vi "ws_mining search for scenario.vi"(6 "User":T3, 7 "httpRequestID":u32, 8 "error in (no error)":errorcluster, 10 "GET (empty)":T1, 11 "Connection Refnum":T2) -> (0 "error out":errorcluster, 1 "Template Keys":T1, 2 "Template":string, 3 "Connection Refnum":T2)   [LabVIEW 2011]
uses:
  server/database/Users/User Record.ctl
  <vilib>/addons/internet/utils/keyedarr.llb/Keyed Array.ctl
  SI.LIB/ODBC/SQL Controls/Connection Refnum.ctl
  <vilib>/addons/internet/utils/strutil.llb/Case Matching.ctl
  <vilib>/wsapi/NI_WebServices.lvlib
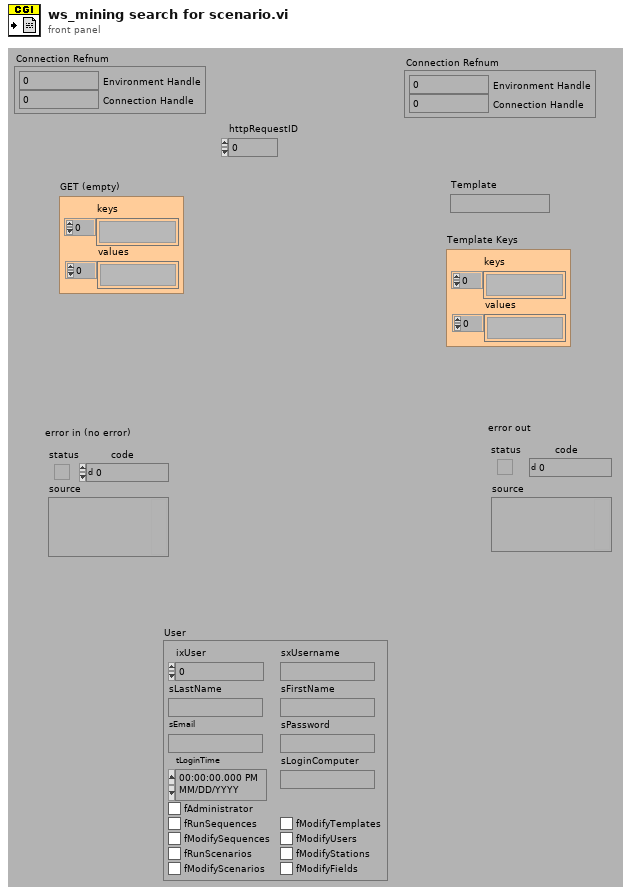
[diagram p1: front panel]
types:
  T1 = typedef "Keyed Array.ctl" = cluster{"keys":string[], "values":string[]}
  T2 = typedef "Connection Refnum.ctl" = cluster{"Environment Handle":i32, "Connection Handle":i32}
  T3 = typedef "User Record.ctl" = cluster{"ixUser":i32, "sxUsername":string, "sLastName":string, "sFirstName":string, "sEmail":string, "sPassword":string, "tLoginTime":timestamp, "sLoginComputer":string, "fAdministrator":bool, "fRunSequences":bool, "fModifySequences":bool, "fRunScenarios":bool, "fModifyScenarios":bool, "fModifyTemplates":bool, "fModifyUsers":bool, "fModifyStations":bool, "fModifyFields":bool}
  T4 = typedef "Case Matching.ctl" = enum16{"a != A", "a == A", "system"}
  T5 = typedef "Scenario Record.ctl" = cluster{"ixScenario":i32, "tCreated":timestamp, "tModified":timestamp, "sxUsername":string, "sModifiedBy":string, "sxScenarioId":string, "sDescription":string, "sLogic":string, "sResultFieldsCSV":string, "sTemplatesCSV":string, "fAutoRunReports":bool, "fSortByTemplates":bool, "fCombinePDF":bool, "Conditions":T6[]}
  T6 = typedef "Condition Record.ctl" = cluster{"iConditionIndex":i32, "sxFieldId":string, "nOperator":T7, "sMatchValue":string}
  T7 = typedef "Condition Operators.ctl" = enum16{"equal (=)", "not equal (\\u2260)", "less than (<)", "less than or equal (\\u2264)", "greater than (>)", "greater than or equal (\\u2265)", "contains", "does not contain"}
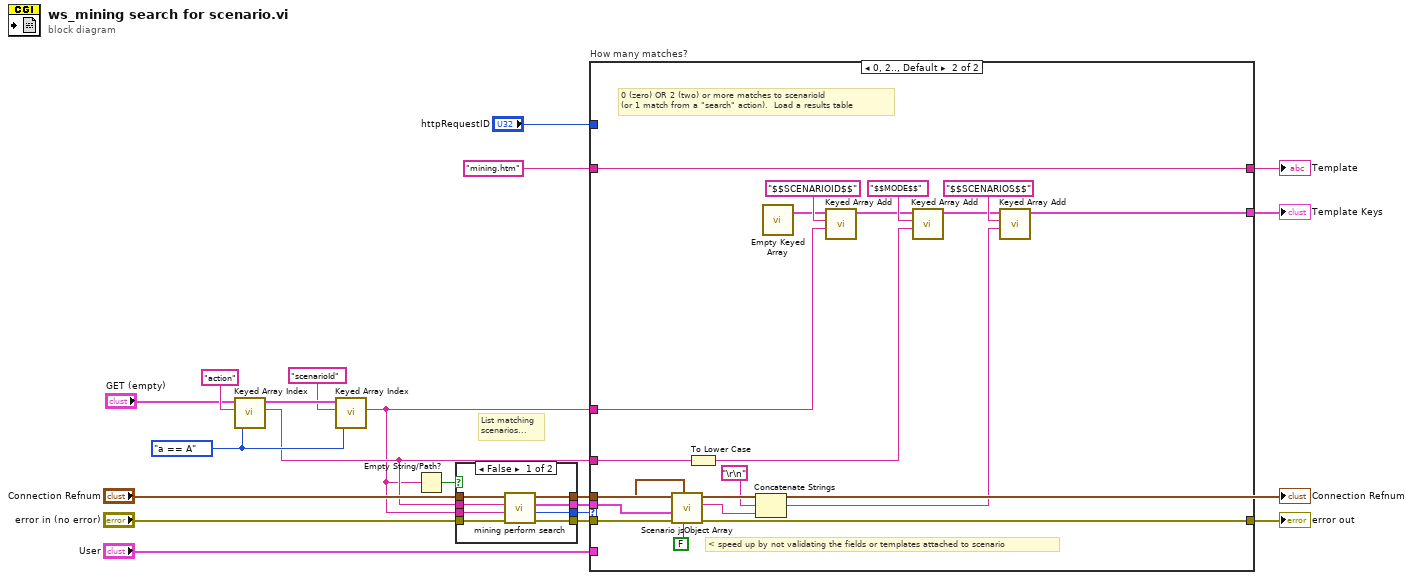
[diagram p0: block diagram]
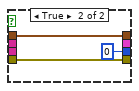
[diagram p2: hidden frame]
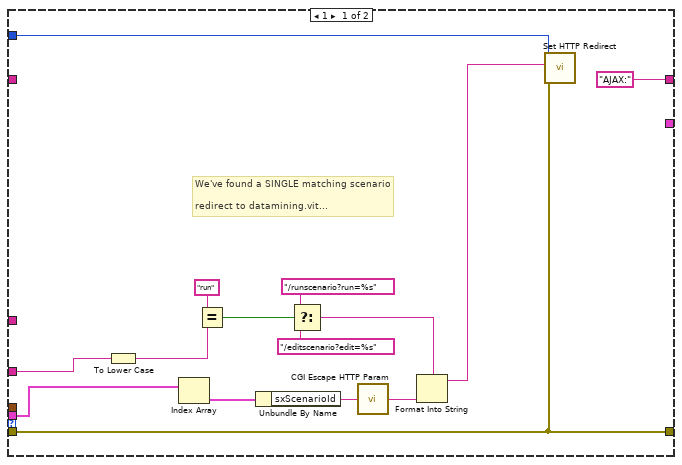
[diagram p3: hidden frame]
diagram:
  w8 = Case_Matching."a == A" ("case matching (sensitive)")
  # "List matching\nscenarios..."
  n1 = call <vilib>:"Keyed Array Index.vi"("case matching (sensitive)"=w8, "key"="action", "array in"="GET (empty)") -> ("value"=w7:string, "duplicate array"=w10:T1)  [unwired: 1 in, 2 out]
  n2 = call <vilib>:"Keyed Array Index.vi"("case matching (sensitive)"=w8, "key"="scenarioId", "array in"=w10) -> ("value"=w4:string)  [unwired: 1 in, 3 out]
  n3 = Empty String/Path?(string/path=w4) -> (empty?=w3:bool)
  n4 = case shown="False" w3 {
    tunnel: "error in (no error)" -> [w28 w30]
    tunnel: "Connection Refnum" -> [w27 w31]
    tunnel: [w26 w31] -> w2
    tunnel: [w25 _] -> w14
    tunnel: [w24 w30] -> w13
    tunnel: w7 -> [w23 _]
    tunnel: [w22 0 ("Matching Results")] -> w5
    tunnel: w4 -> [w21 _]
    frame False {
      n5 = call "mining perform search.vi"("error in (no error)"=w28, "sxScenarioId (\"\")"=w21, "Action (\"Search\")"=w23, "Connection Refnum"=w27) -> ("error out"=w24:errorcluster, "Matching Results"=w22:i32, "Results"=w25:T5[], "Connection Refnum"=w26:T2)  [unwired: 4 out]
    }
    frame True {
    }
  }
  "Connection Refnum" <- w2
  n6 = case "How many matches?" shown="0, 2.., Default" w5 {
    tunnel: w4 -> [_ w50]
    tunnel: w14 -> [w42 w55]
    tunnel: "User" -> [_ _]
    tunnel: [_ w60] -> w20
    tunnel: w13 -> [w33 w57]
    tunnel: [w33 w56] -> w19
    tunnel: ["AJAX:" w64] -> w18
    tunnel: w7 -> [w45 w66]
    tunnel: "httpRequestID" -> [w34 _]
    tunnel: "mining.htm" ("Template (\"\")") -> [_ w64]
    tunnel: w2 -> [_ w49]
    frame 1 {
      # "We've found a SINGLE matching scenario\n\nredirect to datamining.vit..."
      n7 = To Lower Case(string=w45) -> (all lower case string=w43:string)
      n8 = Index Array(array=w42) -> (element=w41:T5)  [unwired: 1 in]
      n9 = Equal?(x="run" ("y"), y=w43) -> (x = y?=w40:bool)
      n10 = Unbundle By Name(w41) -> ("sxScenarioId"=w38:string)
      n11 = Select(t="/runscenario?run=%s" ("New URL (/cgi-bin/testing.vit)"), s=w40, f="/editscenario?edit=%s" ("New URL (/cgi-bin/testing.vit)")) -> (s? t:f=w35:string)
      n12 = call <vilib>:"CGI Escape HTTP Param.vi"("string"=w38) -> ("url-encoded string"=w39:string)
      n13 = Format Into String(format string=w35, w39) -> (resulting string=w32:string)  [unwired: 2 in, 1 out]
      n14 = call <vilib>:"Set HTTP Redirect.vi"("error in (no error)"=w33, "redirect URL"=w32, "httpRequestID"=w34) -> ()  [unwired: 7 in, 2 out]
    }
    frame 0, 2.., Default {
      # "< speed up by not validating the fields or templates attached to scenario"
      # "0 (zero) OR 2 (two) or more matches to scenarioId\n(or 1 match from a \"search\" action).  Load a results table"
      n15 = call "Scenario jsObject Array.vi"("Validate Fields/Templates? (t)"=FALSE, "Connection Refnum"=w49, "error in (no error)"=w57, "SCENARIOS (none)"=w55) -> ("error out"=w56:errorcluster, "Scenarios jsObject Array"=w53:string, "SCENARIOS jsObject Definition"=w54:string)  [unwired: 2 in, 3 out]
      n16 = To Lower Case(string=w66) -> (all lower case string=w58:string)
      n17 = Concatenate Strings(w54, "\r\n", w53) -> (w52:string)
      n18 = call "Empty Keyed Array.vi"() -> ("empty keyed array"=w47:T1)  [unwired: 3 out]
      n19 = call <vilib>:"Keyed Array Add.vi"("value"=w50, "key"="$$SCENARIOID$$", "array in"=w47) -> ("array out"=w59:T1)  [unwired: 2 in, 2 out]
      n20 = call <vilib>:"Keyed Array Add.vi"("value"=w58, "key"="$$MODE$$", "array in"=w59) -> ("array out"=w61:T1)  [unwired: 2 in, 2 out]
      n21 = call <vilib>:"Keyed Array Add.vi"("value"=w52, "key"="$$SCENARIOS$$", "array in"=w61) -> ("array out"=w60:T1)  [unwired: 2 in, 2 out]
    }
  }
  "error out" <- w19
  "Template Keys" <- w20
  "Template" <- w18
